vi "Write Coordinate[].vi"(8 "error in (no error)":errorcluster, 10 "Coordinate[]":T1[](array[typedef]), 11 "TSP Class in":refnum<class "TSP Class.lvclass">) -> (0 "error out":errorcluster, 3 "TSP Class out":refnum<class "TSP Class.lvclass">)   [LabVIEW 2015, in "TSP Library.lvlib" / "TSP Class.lvclass"]
uses:
  TSP Class.lvclass
  TypeDef/Coordinate.ctl
  TSP Class.lvclass/TSP Class.ctl
  TSP Library.lvlib
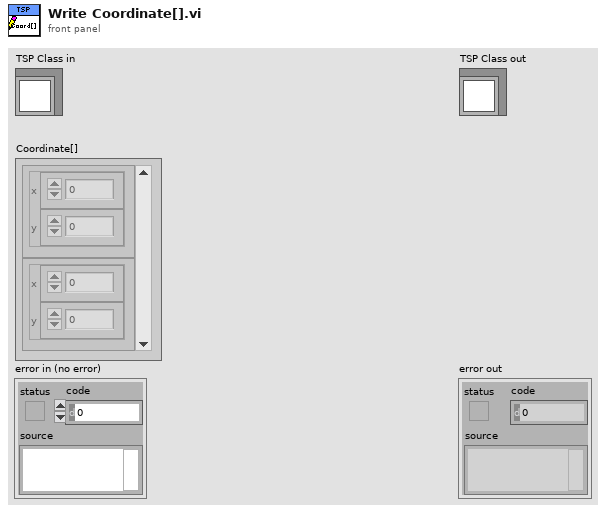
[diagram p1: front panel]
types:
  T1 = typedef "TSP Library.lvlib/Coordinate.ctl" = cluster{"x":dbl, "y":dbl}
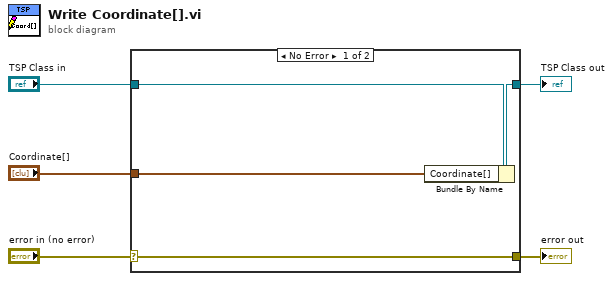
[diagram p0: block diagram]
diagram:
  n1 = case shown="No Error" "error in (no error)" {
    selector: "error in (no error)" -> [w9 w10]
    tunnel: [w9 w10] -> w4
    tunnel: [w7 w11] -> w2
    tunnel: "TSP Class in" -> [w8 w11]
    tunnel: "Coordinate[]" -> [w6 _]
    frame No Error {
      n2 = Bundle By Name(cluster=w8, "Coordinate[]"=w6) -> (w7:refnum<class "TSP Class.lvclass">)
    }
    frame Error {
    }
  }
  "error out" <- w4
  "TSP Class out" <- w2
